vi "Set VISA资源名称.vi"(10 "VISA资源名称":refnum<visa-resource-name>, 11 "GPS in":refnum<class "GPS.lvclass">) -> (3 "GPS out":refnum<class "GPS.lvclass">)   [LabVIEW 2016, in "GPS.lvlib" / "GPS.lvclass"]
uses:
  GPS.lvclass
  GPS.lvclass/GPS.ctl
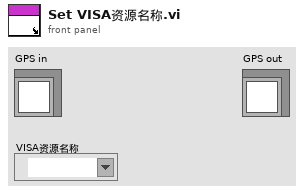
[diagram p1: front panel]
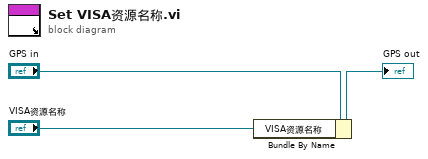
[diagram p0: block diagram]
diagram:
  n1 = Bundle By Name(cluster="GPS in", "VISA资源名称"="VISA资源名称") -> (→"GPS out":refnum<class "GPS.lvclass">)
